vi "Init.vi"() -> (3 "TEMPLATE Msg out":refnum<class "TEMPLATE Msg.lvclass">)   [LabVIEW 2025]
uses:
  TEMPLATE Msg.lvclass/TEMPLATE Msg.ctl
  TEMPLATE Msg.lvclass
panel:
  # "This front panel should not be manipulated."
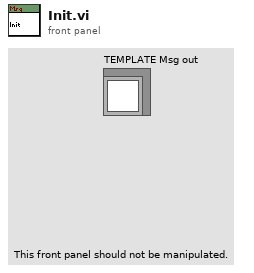
[diagram p1: front panel]
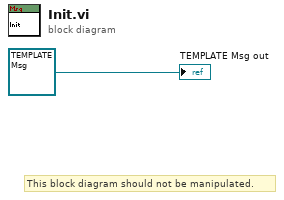
[diagram p0: block diagram]
diagram:
  # "This block diagram should not be manipulated."
  "TEMPLATE Msg out" <- refnum<class "TEMPLATE Msg.lvclass"> refnum ("TEMPLATE Msg out")
